vi "Create Connection Cluster.vi"(9 "instrument_type_id":string, 10 "session":variant, 11 "channel mappings":T3[](array[typedef])) -> (3 "connections":T1[](array[typedef]))   [LabVIEW 2020, in "MeasurementServerTests.lvlib"]
uses:
  MeasurementServerTests.lvlib
  Runtime/MeasurementLink Session Management/Session Reservation/Hardware Independent Connection.ctl
  Runtime/MeasurementLink Session Management/Session Reservation/Session Reservation.lvclass
  Runtime/MeasurementLink Session Management/Session Reservation/Connection.ctl
  Runtime/MeasurementLink Session Management Client/RPC Messages/ni_measurementlink_sessionmanagement_v1_ChannelMapping.ctl
  Runtime/MeasurementLink Session Management Client/MeasurementLink Session Management Client.lvlib
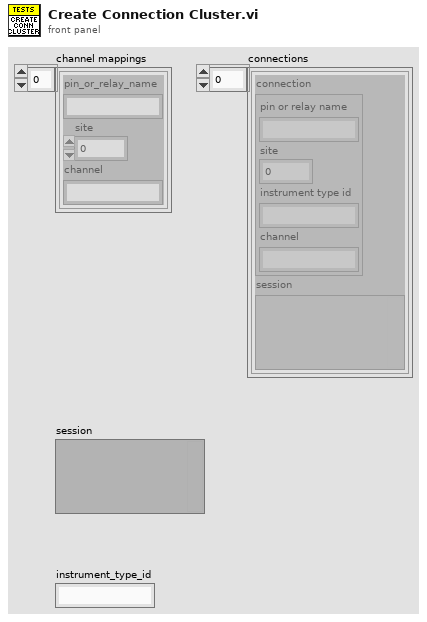
[diagram p1: front panel]
types:
  T1 = typedef "MeasurementLink Session Management.lvlib/Session Reservation.lvclass/Connection.ctl" = cluster{"connection":T2, "session":variant}
  T2 = typedef "MeasurementLink Session Management.lvlib/Session Reservation.lvclass/Hardware Independent Connection.ctl" = cluster{"pin or relay name":string, "site":i32, "instrument type id":string, "channel":string}
  T3 = typedef "MeasurementLink Session Management Client.lvlib/ni_measurementlink_sessionmanagement_v1_ChannelMapping.ctl" = cluster{"pin_or_relay_name":string, "site":i32, "channel":string}
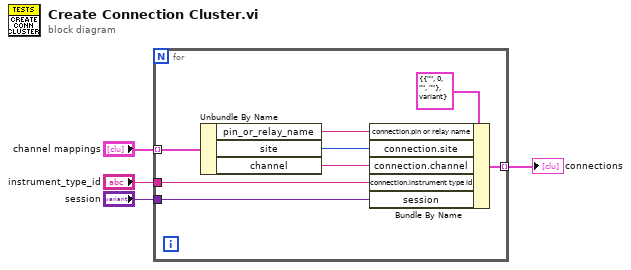
[diagram p0: block diagram]
diagram:
  n1 = for {
    tunnel: [w10] -> w4 mode=indexing
    tunnel: "session" -> [w9]
    tunnel: "instrument_type_id" -> [w6]
    tunnel: "channel mappings" -> [w5] mode=indexing
    n2 = Unbundle By Name(w5) -> ("pin_or_relay_name"=w11:string, "site"=w12:i32, "channel"=w7:string)
    n3 = Bundle By Name(cluster=T1 {"connection"={"pin or relay name"="", "site"=0, "instrument type id"="", "channel"=""}, "session"=variant} ("connection"), "connection.pin or relay name"=w11, "connection.site"=w12, "connection.channel"=w7, "connection.instrument type id"=w6, "session"=w9) -> (w10:T1)
  }
  "connections" <- w4
